vi "Get path.vi"(10 "File mame":path, 11 "VI in":refnum<vi>) -> (3 "File path":path)   [LabVIEW 2023]
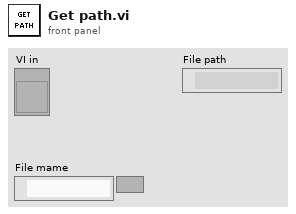
[diagram p1: front panel]
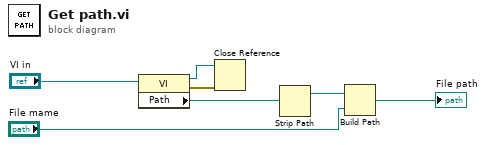
[diagram p0: block diagram]
diagram:
  n1 = property class="VI"(reference="VI in") -> (reference out=w3:refnum<vi>, error out=w2:errorcluster, "Path"=w4:path)  [unwired: 1 in]
  n2 = Close Reference(reference=w3, error in (no error)=w2) -> ()  [unwired: 1 out]
  n3 = Strip Path(path=w4) -> (stripped path=w5:path)  [unwired: 1 out]
  n4 = Build Path(base path=w5, name or relative path="File mame") -> (appended path=→"File path":path)
